vi "send_receive_command.vi"(0 "reference (in)":refnum<class "_Controller.lvclass">, 2 "ASCII Command (in)":string, 5 "error in (no error)":errorcluster) -> (14 "reference (out)":refnum<class "_Controller.lvclass">, 16 "response (out)":string, 17 "write_string (out)":string="ID", 18 "success?":bool, 19 "error out":errorcluster)   [LabVIEW 2013, in "classes.lvlib" / "_Controller.lvclass"]
doc: "Takes as input a controller reference and an ASCII command input (refer to the ASCII Language Specification of the USB Communication API documenation for permissible commands for the referenced controller). The reference input (and passed through as an output) is an instantiated Class reference for the attached controller. Implementss the USB Communication API function \"fnPerformaxComSendRecv\". \n\nProduced By:\n\n<B>Kod Integrations, LLC</B>\n4835 Marianne Drive\nMount Airy, MD 21771\nhttp://www.kodintegrations.com\nemail: info@kodintegrations.com\nphone: (240) 687-1288"
uses:
  _Controller.lvclass
  translate_to_from_byte_array_actions.ctl
  _Controller.lvclass/_Controller.ctl
  error_actions.ctl
  common.lvlib
  PerformaxCom.dll
panel:
  in  "pre_init_bytearray (hidden)":u8[](array[numeric])=[0, 0, 0, 0, 0, 0, 0, 0, 0, 0, 0, 0, 0, 0, 0, 0, 0, 0, 0, 0, 0, 0, 0, 0, 0, 0, 0, 0, 0, 0, 0, 0, 0, 0, 0, 0, 0, 0, 0, 0, 0, 0, 0, 0, 0, 0, 0, 0, 0, 0, 0, 0, 0, 0, 0, 0, 0, 0, 0, 0, 0, 0, 0, 0]
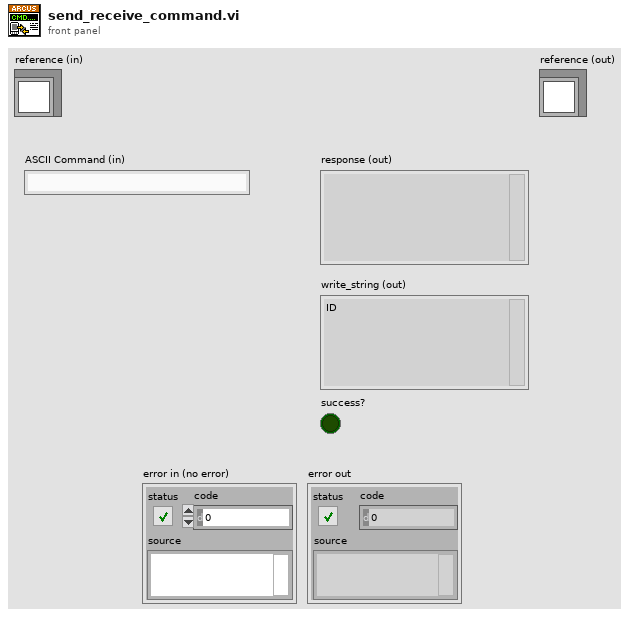
[diagram p1: front panel]
types:
  T1 = typedef "common.lvlib/translate_to_from_byte_array_actions.ctl" = enum16{"to_bytes", "to_string"}
  T2 = typedef "common.lvlib/error_actions.ctl" = enum16{"clearBuff", "closeRef", "nodeErr", "noDeviceInfo", "noDevices", "openRef", "sendReceive", "setTimeouts", "unknown"}
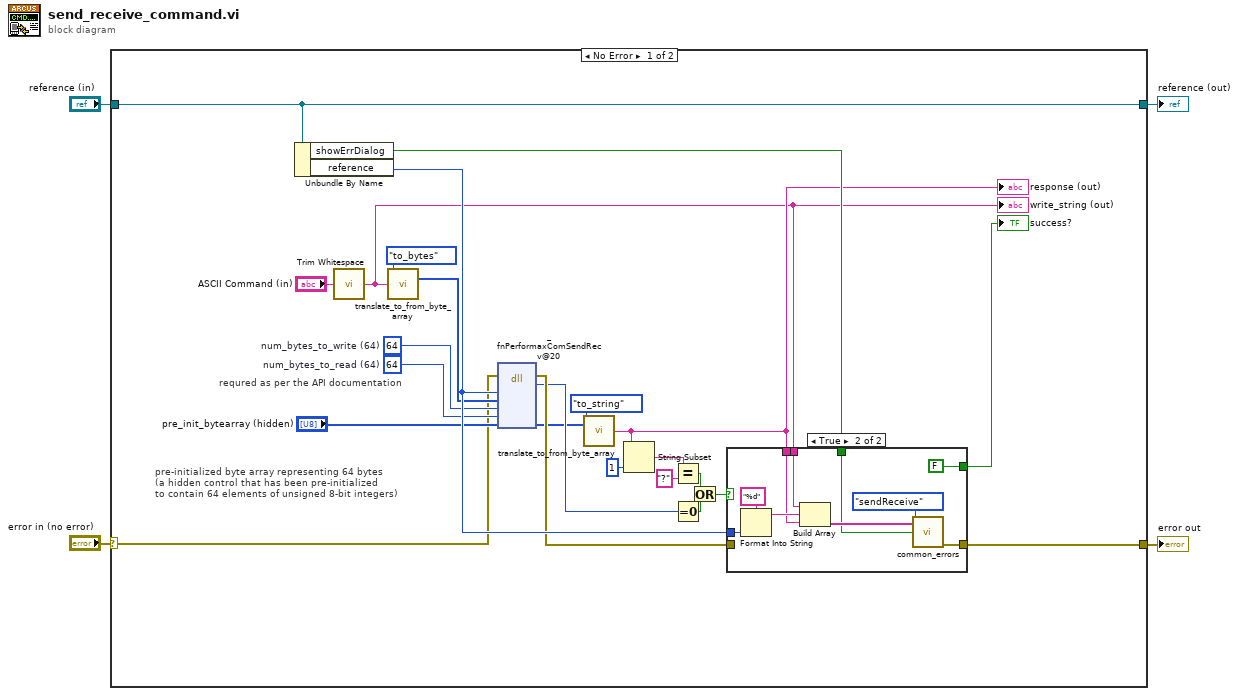
[diagram p0: block diagram]
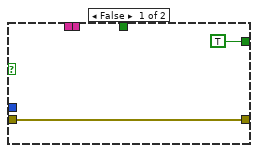
[diagram p2: hidden frame]
diagram:
  n1 = case shown="No Error" "error in (no error)" {
    selector: "error in (no error)" -> [w7 w41]
    tunnel: "reference (in)" -> [w5 w42]
    tunnel: [w6 w41] -> w2
    tunnel: [w5 w42] -> w1
    frame No Error {
      w12 = 64  # num_bytes_to_write (64)
      w13 = 64  # num_bytes_to_read (64)
      # "requred as per the API documentation"
      # "pre-initialized byte array representing 64 bytes\n(a hidden control that has been pre-initialized\nto contain 64 elements of unsigned 8-bit integers)"
      n2 = Unbundle By Name(w5) -> ("showErrDialog"=w27:bool, "reference"=w26:i32)
      n3 = call "Trim Whitespace.vi"("string"="ASCII Command (in)") -> ("trimmed string"=w14:string)  [unwired: 1 in]
      "write_string (out)" <- w14
      n4 = call "translate_to_from_byte_array.vi"("actions"=translate_to_from_byte_array_actions."to_bytes", "string (in)"=w14) -> ("byte_array (out)"=w9:u8[])  [unwired: 12 in, 1 out]
      n5 = dll-call lib="C:/Program Files (x86)/Arcus Technology/Drivers, Libraries, Source/Performax USB v4.01/PerformaxCom.dll" fn="_fnPerformaxComSendRecv@20"(error in=w7, "reference"=w26, "writeBuffer"=w9, "numBytesToWrite"=w12, "numBytesToRead"=w13, "readBuffer"="pre_init_bytearray (hidden)") -> (error out=w22:errorcluster, "return type"=w15:i32, "readBuffer"=w8:u8[])  [unwired: 6 in, 1 out]
      n6 = call "translate_to_from_byte_array.vi"("actions"=translate_to_from_byte_array_actions."to_string", "byte_array (in)"=w8) -> ("string (out)"=w24:string)  [unwired: 12 in, 1 out]
      "response (out)" <- w24
      n7 = String Subset(string=w24, length (rest)=1 ("length (rest)")) -> (substring=w21:string)  [unwired: 1 in]
      n8 = Equal?(x=w21, y="?") -> (x = y?=w17:bool)
      n9 = Equal To 0?(x=w15) -> (x = 0?=w18:bool)
      n10 = Or(x=w17, y=w18) -> (x .or. y?=w19:bool)
      n11 = case shown="True" w19 {
        tunnel: [w30 w39] -> w6
        tunnel: w22 -> [w30 _]
        tunnel: w26 -> [_ w36]
        tunnel: w14 -> [_ w34]
        tunnel: [TRUE FALSE] -> w23
        tunnel: w24 -> [_ w32]
        tunnel: w27 -> [_ w31]
        frame False {
        }
        frame True {
          n12 = Format Into String(format string="%d", w36) -> (resulting string=w35:string)  [unwired: 2 in, 1 out]
          n13 = Build Array(w34, w35, w32) -> (w37:string[])
          n14 = call "common_errors.vi"("common_errors"=error_actions."sendReceive" ("errors"), "dialog? (T)"=w31, "supp_text"=w37) -> ("error out"=w39:errorcluster)  [unwired: 12 in]
        }
      }
      "success?" <- w23
    }
    frame Error {
    }
  }
  "error out" <- w2
  "reference (out)" <- w1
